vi "ENPH354_LabLightMeter.vi"() -> ()   [LabVIEW 2020]
uses:
  <vilib>/MakerHub/LINX/Public/Peripherals/PWM/PWM Set Duty Cycle 1 Chan.vi
  <vilib>/MakerHub/LINX/Public/Peripherals/Analog/Analog Read 1 Chan.vi
  <vilib>/MakerHub/LINX/Public/Peripherals/Digital/Digital Write N Chans.vi
  <vilib>/Analysis/baseanly.llb/Mean (DBL).vi
  <vilib>/MakerHub/LINX/Public/Peripherals/Analog/Analog Read N Chans.vi
  <vilib>/MakerHub/LINX/Private/Local IO/LinxDigitalWrite.vi
  <vilib>/MakerHub/LINX/Public/Utilities/Check Channel.vi
  <vilib>/MakerHub/LINX/Private/Local IO/LinxAnalogRead.vi
  <vilib>/MakerHub/LINX/Public/Utilities/Open Serial.vi
  <vilib>/MakerHub/LINX/Public/Peripherals/PWM/PWM Set Duty Cycle N Chans.vi
  <vilib>/MakerHub/LINX/Private/Utilties/Generate Error.vi
  <vilib>/MakerHub/LINX/LMH-LINX.lvlib
  <vilib>/Analysis/NI_AALBase.lvlib
panel:
  out "error out":errorcluster
  out "Real Time Mean":dbl
  in  "Use Knob":bool
  out "Duty Cycle":dbl
  out "Averaged V vs Duty-Cycle":cluster{"X":dbl[], "Y":dbl[]}[](graph)
  in  "Knob":dbl(knob) scale=0.0..1.0
  in  "stop":bool
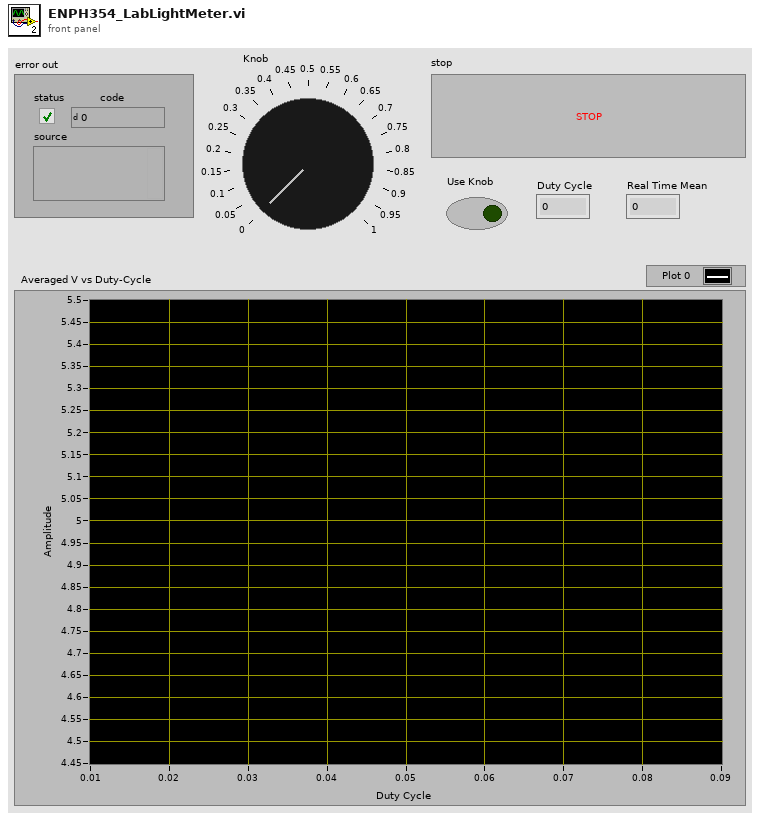
[diagram p1: front panel]
types:
  T1 = typedef "LMH-LINX.lvlib/LINX Ref.ctl" = cluster{"IO":T2, "Interface":T3, "LINX Device Config":T4}
  T2 = typedef "LMH-LINX.lvlib/Platform.ctl" = enum16{"Remote", "Local"}
  T3 = typedef "LMH-LINX.lvlib/Interface.ctl" = enum16{"Serial", "TCP"}
  T4 = typedef "LMH-LINX.lvlib/Device.lvlib/LINX Device Config.ctl" = cluster{"Interface":T3, "COM Port":refnum<visa-resource-name>, "TCP Configuration":T5, "Device Family":u8, "Device ID":u8, "Device Name":string, "TCP Ref":refnum<k5>, "Channels":T6}
  T5 = typedef "LMH-LINX.lvlib/Device.lvlib/TCP Config.ctl" = cluster{"IP Address":string, "Port":u16}
  T6 = typedef "LMH-LINX.lvlib/Channels.ctl" = cluster{"DI":u8[], "DO":u8[], "AI":u8[], "AO":u8[], "PWM":u8[], "QE":u8[], "UART":u8[], "I2C 2":u8[], "SPI":u8[], "CAN":u8[], "Servo":u8[], "AI Ref (V)":dbl, "AI Resolution (Bits)":u8, "AO Ref (V)":dbl, "AO Resolution (Bits)":u8}
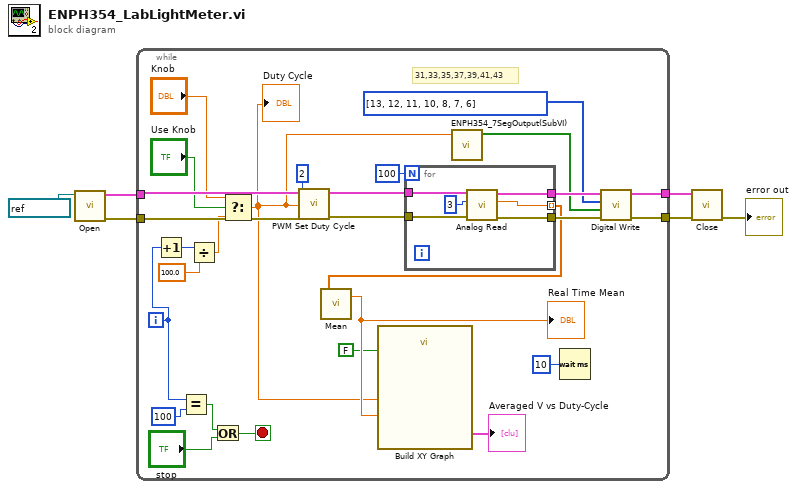
[diagram p0: block diagram]
diagram:
  n1 = call-poly <vilib>:"Open.vi"("Serial Port"=refnum<visa-resource-name> "COM4") -> ("Error Out"=w4:errorcluster, "LINX Resource"=w5:T1)  [unwired: 8 in, 1 out]
  n2 = while {
    tunnel: w5 -> [w34]
    tunnel: w4 -> [w33]
    tunnel: [w13] -> w3
    tunnel: [w12] -> w2
    i -> [w11]
    stop <- w7 stop-if-true
    # "31,33,35,37,39,41,43"
    n3 = Increment(x=w11) -> (x+1=w28:i32)
    n4 = Equal?(x=w11, y=100) -> (x = y?=w9:bool)
    n5 = Divide(x=w28, y=100.0) -> (x/y=w22:dbl)
    n6 = Or(x=w9, y="stop") -> (x .or. y?=w7:bool)
    n7 = Select(t="Knob", s="Use Knob", f=w22) -> (s? t:f=w15:dbl)
    "Duty Cycle" <- w15
    n8 = call-poly <vilib>:"PWM Set Duty Cycle.vi"("Error In"=w33, "Duty Cycle (0-1)"=w15, "PWM Channel"=u8 2, "LINX Resource"=w34) -> ("Error Out"=w30:errorcluster, "LINX Resource"=w31:T1)  [unwired: 6 in]
    n9 = for {
      N: 100 -> [_]
      tunnel: w31 -> [w40]
      tunnel: w30 -> [w39]
      tunnel: [w37] -> w20 mode=indexing
      tunnel: [w36] -> w26
      tunnel: [w35] -> w25
      n10 = call-poly <vilib>:"Analog Read.vi"("Error In"=w39, "Analog Channel"=u8 3, "LINX Resource"=w40) -> ("Error Out"=w35:errorcluster, "Voltage"=w37:dbl, "LINX Resource"=w36:T1)  [unwired: 5 in, 1 out]
    }
    n11 = call-poly <vilib>:"Mean.vi"("X"=w20) -> ("mean"=w19:dbl)  [unwired: 1 out]
    "Real Time Mean" <- w19
    n12 = call "Build XY Graph"("Reset"=FALSE, "Y Input"=w19, "X Input"=w15) -> ("XY Graph"=→"Averaged V vs Duty-Cycle":cluster{"X":dbl[], "Y":dbl[]}[])  [unwired: 7 in, 1 out]
    n13 = call "ENPH354_7SegOutput(SubVI).vi"("Knob"=w15) -> ("Array"=w16:bool[])  [unwired: 10 in]
    n14 = Wait (ms)(milliseconds to wait=u32 10) -> ()  [unwired: 1 out]
    n15 = call-poly <vilib>:"Digital Write.vi"("Error In"=w25, "Values"=w16, "DO Channels"=u8[] [13, 12, 11, 10, 8, 7, 6], "LINX Resource"=w26) -> ("Error Out"=w12:errorcluster, "LINX Resource"=w13:T1)  [unwired: 6 in]
  }
  n16 = call <vilib>:"Close.vi"("Error In"=w2, "LINX Resource"=w3) -> ("Error Out"=→"error out":errorcluster)  [unwired: 9 in]
